vi "AlGaInPAs_v21e.vi"(2 "Debug Mode":bool, 3 "Elapsed Time(s)":dbl, 4 "State":enum16{"Edit", "Start", "Run", "End", "Idle"}(ring), 5 "Argument List In":string[](array[string])) -> (0 "Status Out":string, 1 "Argument List Out":string[](array[string]))   [LabVIEW 2011]
uses:
  high_level_proc/source_noDilute.ctl
  high_level_proc/source_noDilution.ctl
panel:
  in  "Zn bubbler":T1={"Dilution"=FALSE, "Calculated"=0, "MFC1 flow"=0.0, "MFC2 flow"=10.0, "MFC3 flow"=100.0, "Bubbler (main)"={"Flow"=0.0, "Prep"=FALSE, "Run"=FALSE, "Active"=FALSE, "Name"=""}} caption="Al" {"Bubbler (main)"."Flow" format="%.2f"; "MFC1 flow" format="%.4f"; "MFC3 flow" format="%.1f"; "MFC2 flow" format="%.2f"; "Calculated" items=["Flow", "MFC1", "MFC2", "MFC3"]}
  in  "Array":refnum<vi>[](array[refnum])
  in  "Al bubbler":T2 caption="Al" {"Flow" format="%.2f"}
  in  "Se bubbler":T1={"Dilution"=FALSE, "Calculated"=0, "MFC1 flow"=0.0, "MFC2 flow"=10.0, "MFC3 flow"=100.0, "Bubbler (main)"={"Flow"=0.0, "Prep"=FALSE, "Run"=FALSE, "Active"=FALSE, "Name"=""}} caption="Al" {"Bubbler (main)"."Flow" format="%.2f"; "MFC1 flow" format="%.4f"; "MFC3 flow" format="%.1f"; "MFC2 flow" format="%.2f"; "Calculated" items=["Flow", "MFC1", "MFC2", "MFC3"]}
  in  "P bubbler":T2 caption="Al" {"Flow" format="%.2f"}
  in  "As gas":T2 caption="Al" {"Flow" format="%.2f"}
  in  "P gas":T2 caption="Al" {"Flow" format="%.2f"}
  in  "In bubbler":T2 caption="Al" {"Flow" format="%.2f"}
  in  "Tab Control":T3(tab)
  out "Al Prep":bool caption="Pre-run"
  out "Al Run":bool caption="Run"
  out "Al Flow":dbl caption="Al Flow (0-100 sscm)" format="%.2f"
  out "Ga MFC1 flow":dbl caption="R1 (0-10 sscm)" format="%.4f"
  out "Ga MFC3 flow":dbl=100.0 caption="R3 (0-1000 sscm)" format="%.1f"
  out "Ga MFC2 flow":dbl=10.0 caption="R2 (0-100 sscm)" format="%.2f"
  out "Ga Calculated":u16(ring)=1 caption="Calculated" items=["Ga flow", "MFC1", "MFC2", "MFC3"]
  out "Ga Dilution":bool caption="Dilute"
  out "Ga Prep":bool caption="Pre-run"
  out "Ga Run":bool caption="Run"
  out "Ga Flow":dbl caption="Ga Flow (0-10 sscm)" format="%.2f"
  out "In Prep":bool caption="Pre-run"
  out "In Run":bool caption="Run"
  out "In Flow":dbl caption="In Flow (0-100 sscm)" format="%.2f"
  out "P gas Run":bool caption="Run"
  out "P gas Prep":bool caption="Pre-run"
  out "P gas Flow":dbl caption="PH3 Flow (0-100 sscm)" format="%.2f"
  out "As gas Prep":bool caption="Pre-run"
  out "As gas Run":bool caption="Run"
  out "As gas Flow":dbl caption="AsH3 Flow (0-10 sscm)" format="%.2f"
  out "P liq Prep":bool caption="Pre-run"
  out "P liq Run":bool caption="Run"
  out "P liq Flow":dbl caption="P bubbler Flow (0-100 sscm)" format="%.2f"
  out "Zn Flow":dbl caption="Zn Flow (0-10 sscm)" format="%.2f"
  out "Zn Run":bool caption="Run"
  out "Zn Prep":bool caption="Pre-run"
  out "Zn  Dilution":bool caption="Dilute"
  out "Zn Calculated":u16(ring)=1 caption="Calculated" items=["Ga flow", "MFC1", "MFC2", "MFC3"]
  out "Zn MFC2 flow":dbl=10.0 caption="R2 (0-100 sscm)" format="%.2f"
  out "Zn MFC3 flow":dbl=100.0 caption="R3 (0-1000 sscm)" format="%.1f"
  out "Zn MFC1 flow":dbl caption="R1 (0-10 sscm)" format="%.4f"
  out "Se MFC1 flow":dbl caption="R1 (0-10 sscm)" format="%.4f"
  out "Se MFC3 flow":dbl=100.0 caption="R3 (0-1000 sscm)" format="%.1f"
  out "Se MFC2 flow":dbl=10.0 caption="R2 (0-100 sscm)" format="%.2f"
  out "Se Calculated":u16(ring)=1 caption="Calculated" items=["Ga flow", "MFC1", "MFC2", "MFC3"]
  out "Se Dilution":bool caption="Dilute"
  out "Se Prep":bool caption="Pre-run"
  out "Se Run":bool caption="Run"
  out "Se Flow":dbl caption="Se Flow (0-10 sscm)" format="%.2f"
  in  "Ga bubbler":T1={"Dilution"=FALSE, "Calculated"=0, "MFC1 flow"=0.0, "MFC2 flow"=10.0, "MFC3 flow"=100.0, "Bubbler (main)"={"Flow"=0.0, "Prep"=FALSE, "Run"=FALSE, "Active"=FALSE, "Name"=""}} caption="Al" {"Bubbler (main)"."Flow" format="%.2f"; "MFC1 flow" format="%.4f"; "MFC3 flow" format="%.1f"; "MFC2 flow" format="%.2f"; "Calculated" items=["Flow", "MFC1", "MFC2", "MFC3"]}
  out "prep_done":bool
  out "run started":bool
  out "first":bool=TRUE
  out "total time":dbl
  out "is OK?":bool
  in  "prep_time":dbl
  in  "Cancel":bool
  in  "OK":bool
  out "tTotal(s) 2":dbl
  # "s"
  # "Add pre-run time to run time in editor."
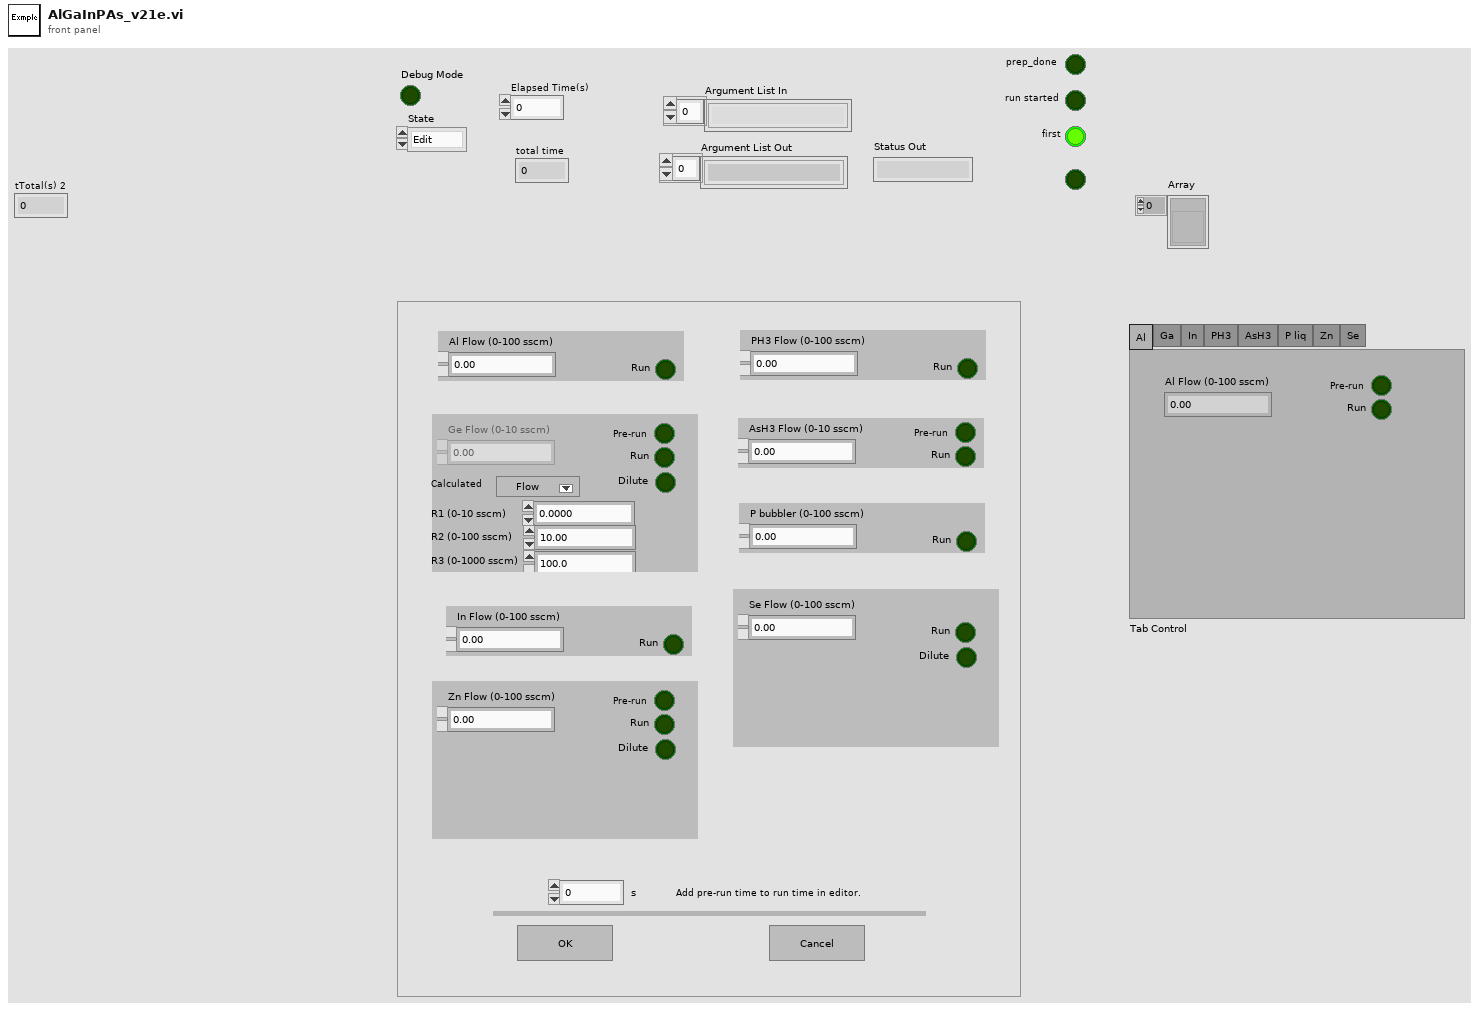
[diagram p1: front panel]
types:
  T1 = typedef "source_noDilute.ctl" = cluster{"Dilution":bool, "Calculated":u16, "MFC1 flow":dbl, "MFC2 flow":dbl, "MFC3 flow":dbl, "Bubbler (main)":T2}
  T2 = typedef "source_noDilution.ctl" = cluster{"Flow":dbl, "Prep":bool, "Run":bool, "Active":bool, "Name":string}
  T3 = enum32{"Al", "Ga", "In", "PH3", "AsH3", "P liq", "Zn", "Se"}
  T4 = enum16{"Discrete", "Continuous", "Instantaneous", "Finite"}
  T5 = enum32{"Invalid", "Default", "Floating", "Floating/Auto-Hide", "Modal"}
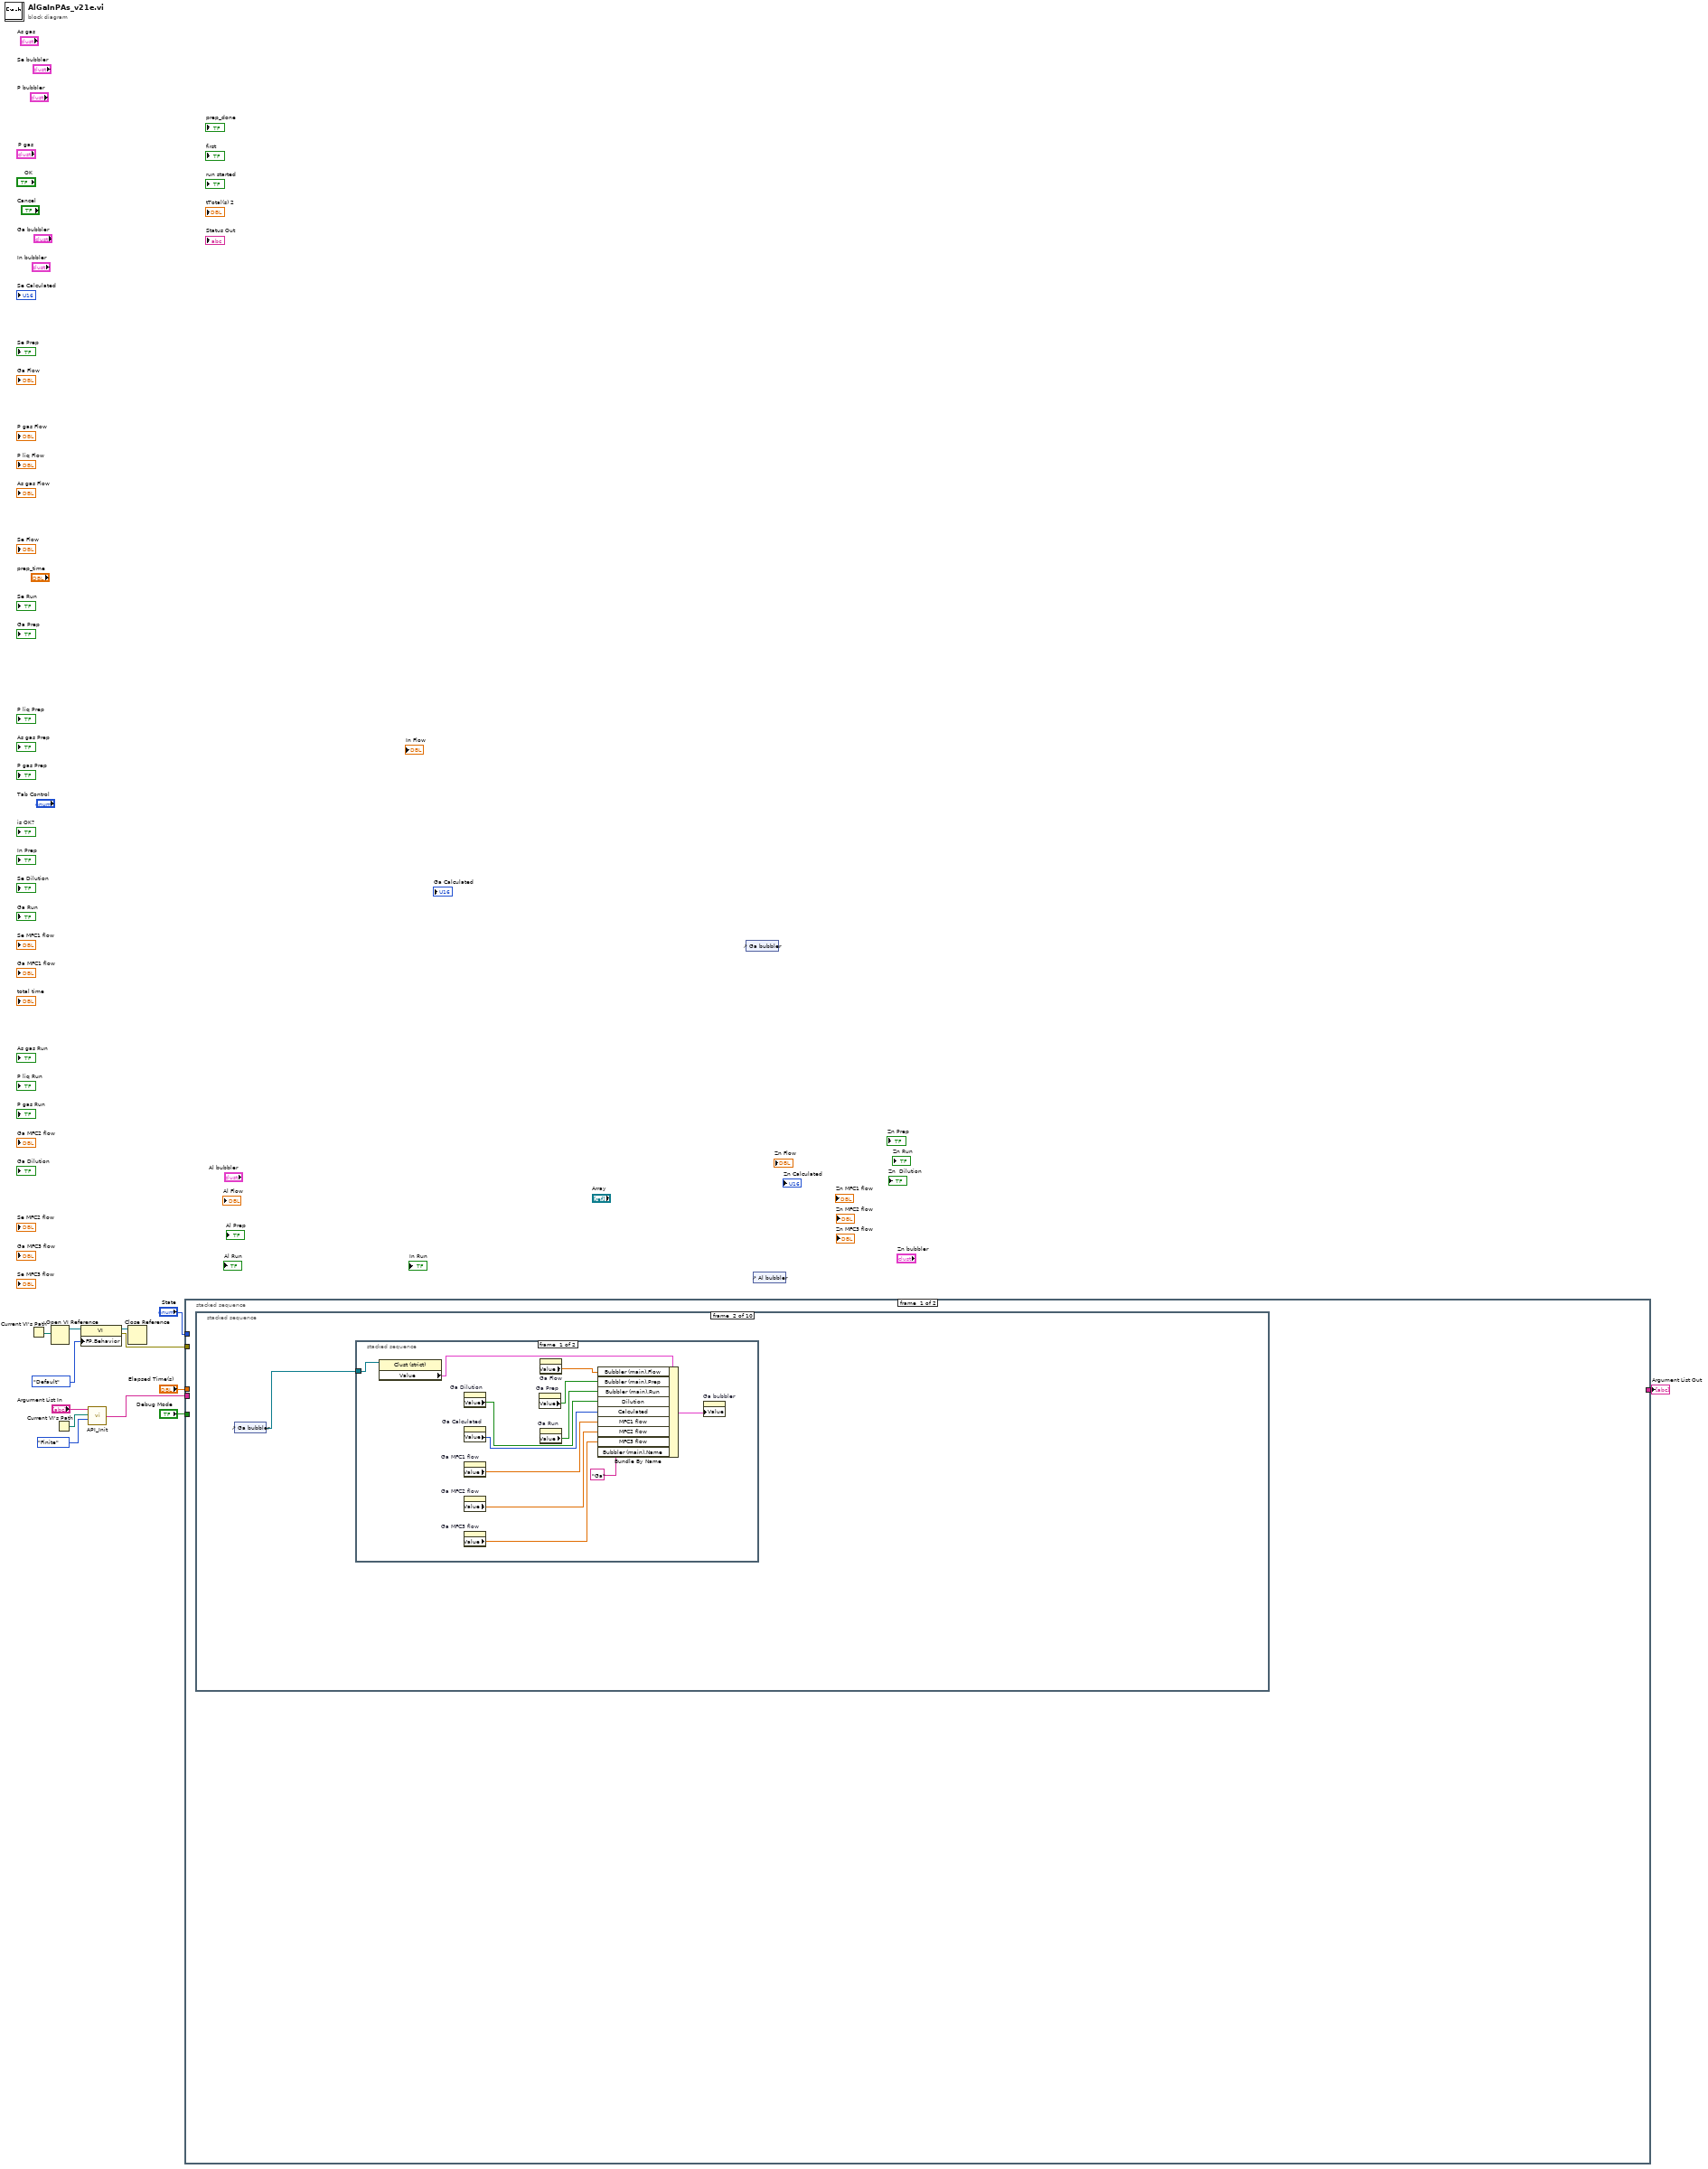
[diagram p0: block diagram]
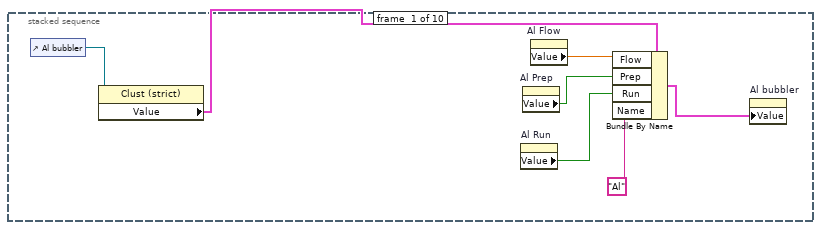
[diagram p2: hidden frame]
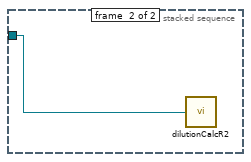
[diagram p3: hidden frame]
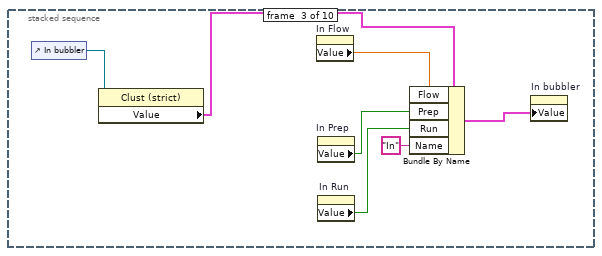
[diagram p4: hidden frame]
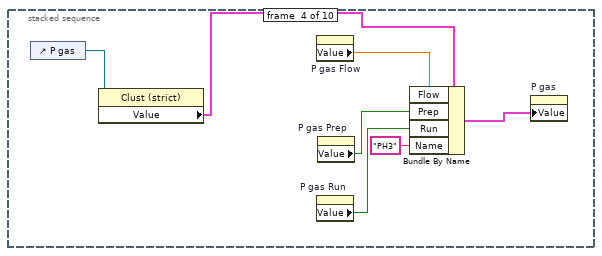
[diagram p5: hidden frame]
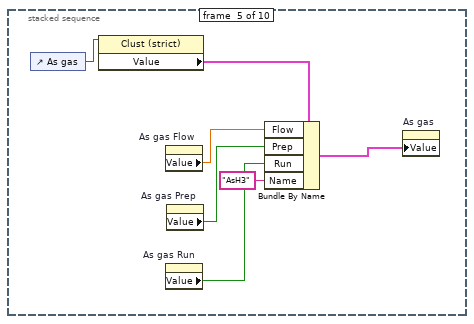
[diagram p6: hidden frame]
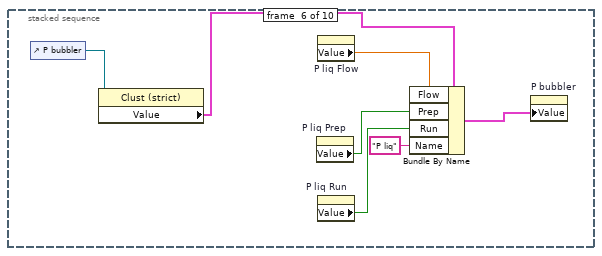
[diagram p7: hidden frame]
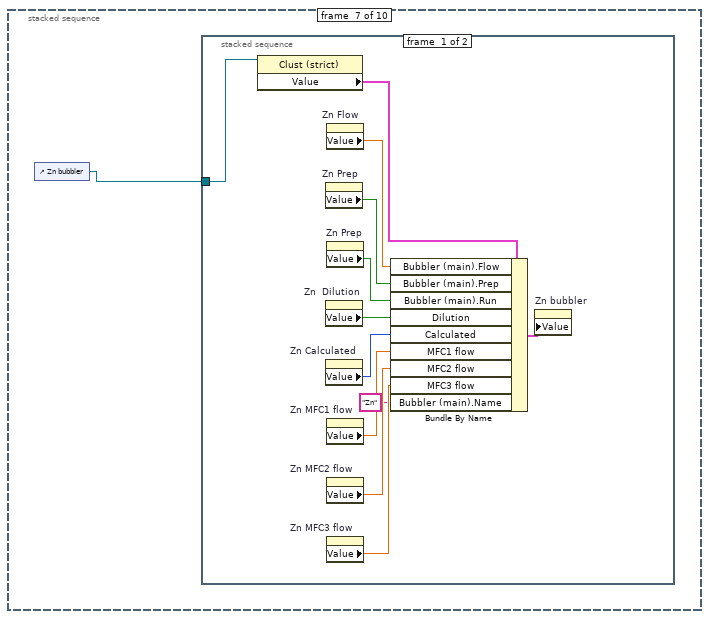
[diagram p8: hidden frame]
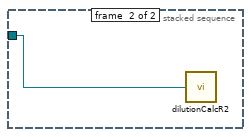
[diagram p9: hidden frame]
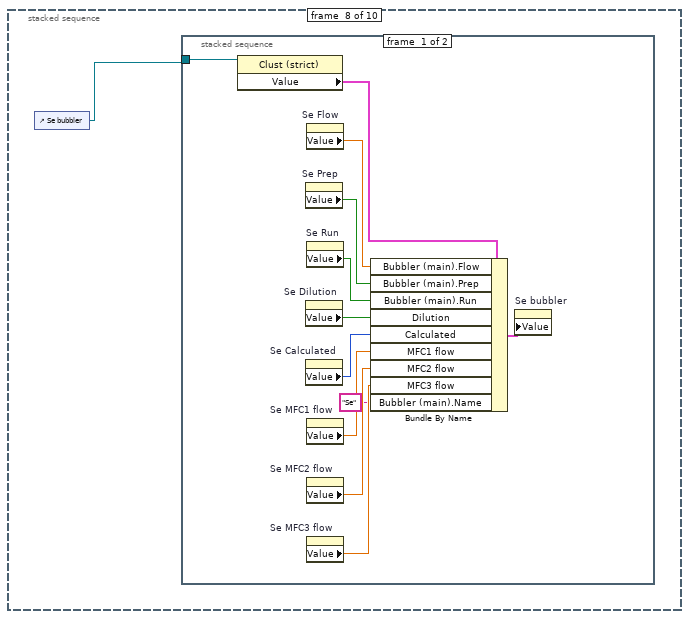
[diagram p10: hidden frame]
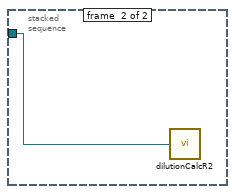
[diagram p11: hidden frame]
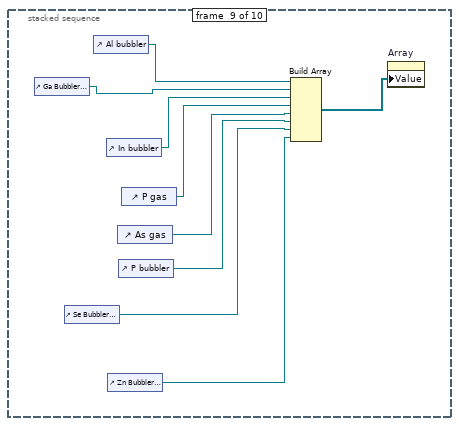
[diagram p12: hidden frame]
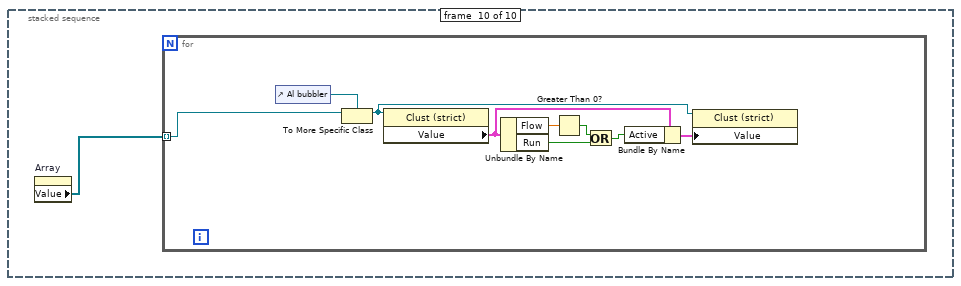
[diagram p13: hidden frame]
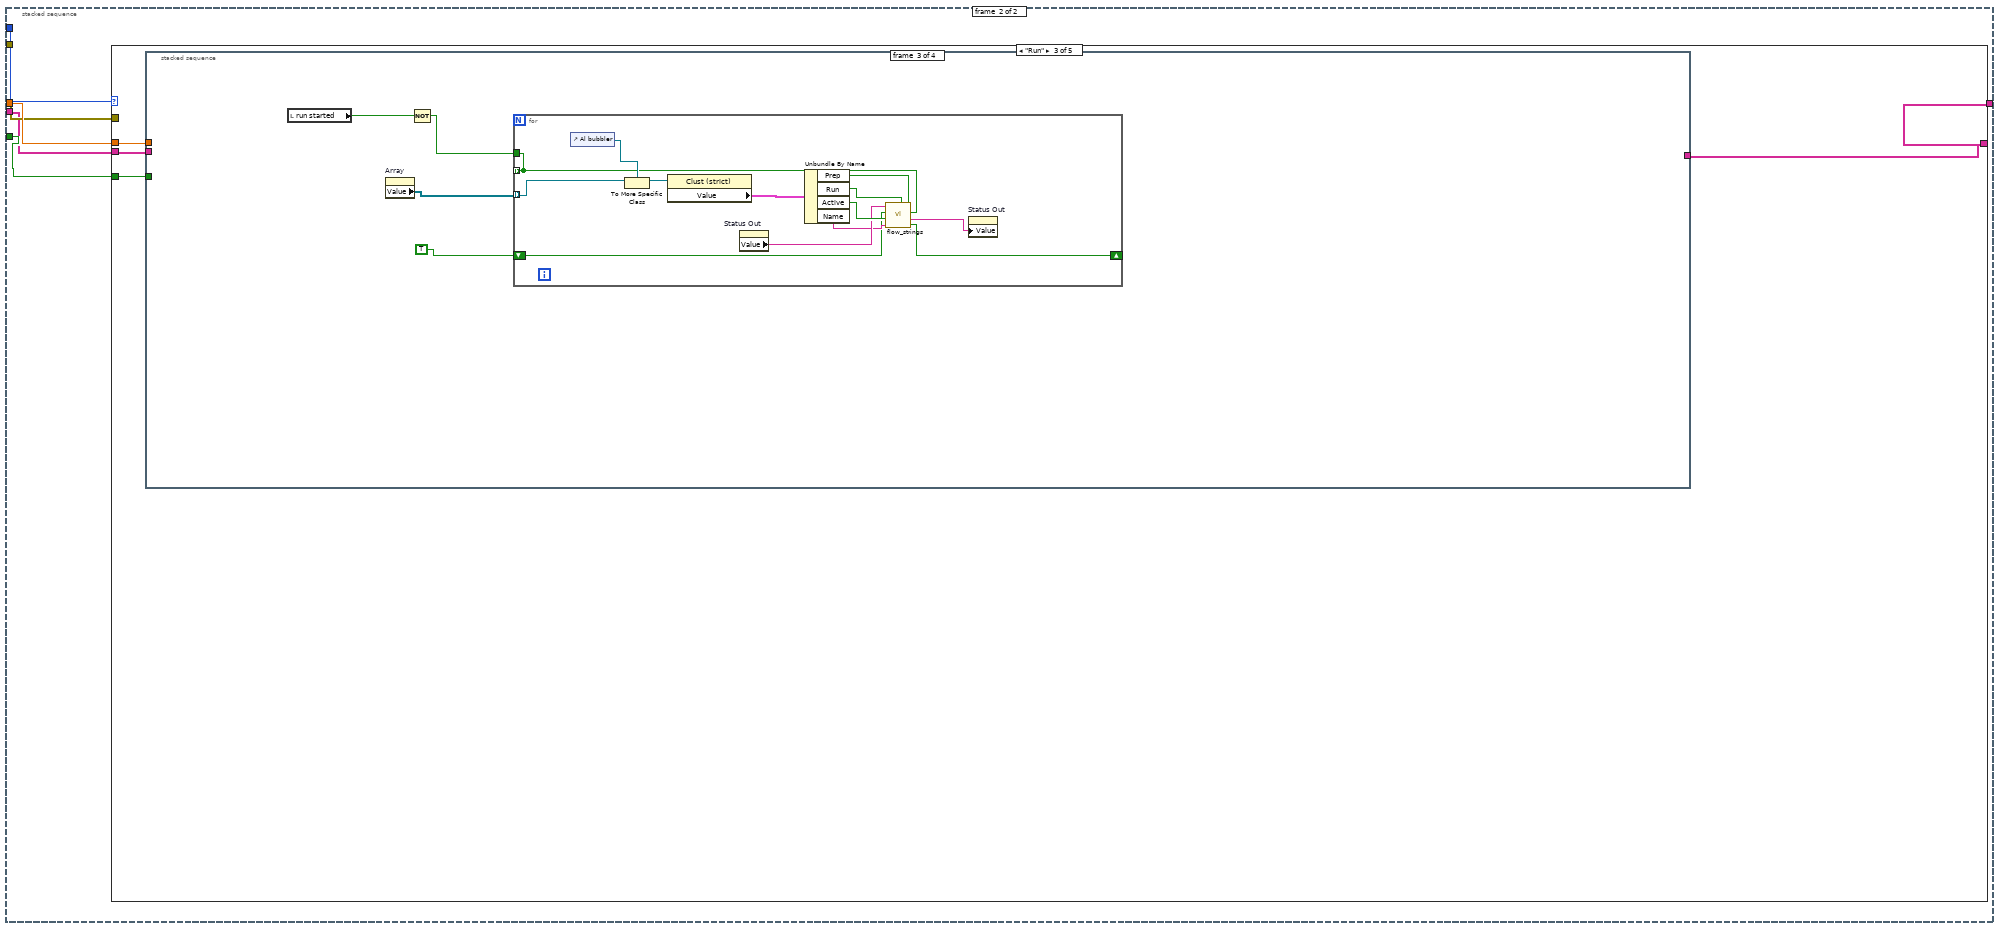
[diagram p14: hidden frame]
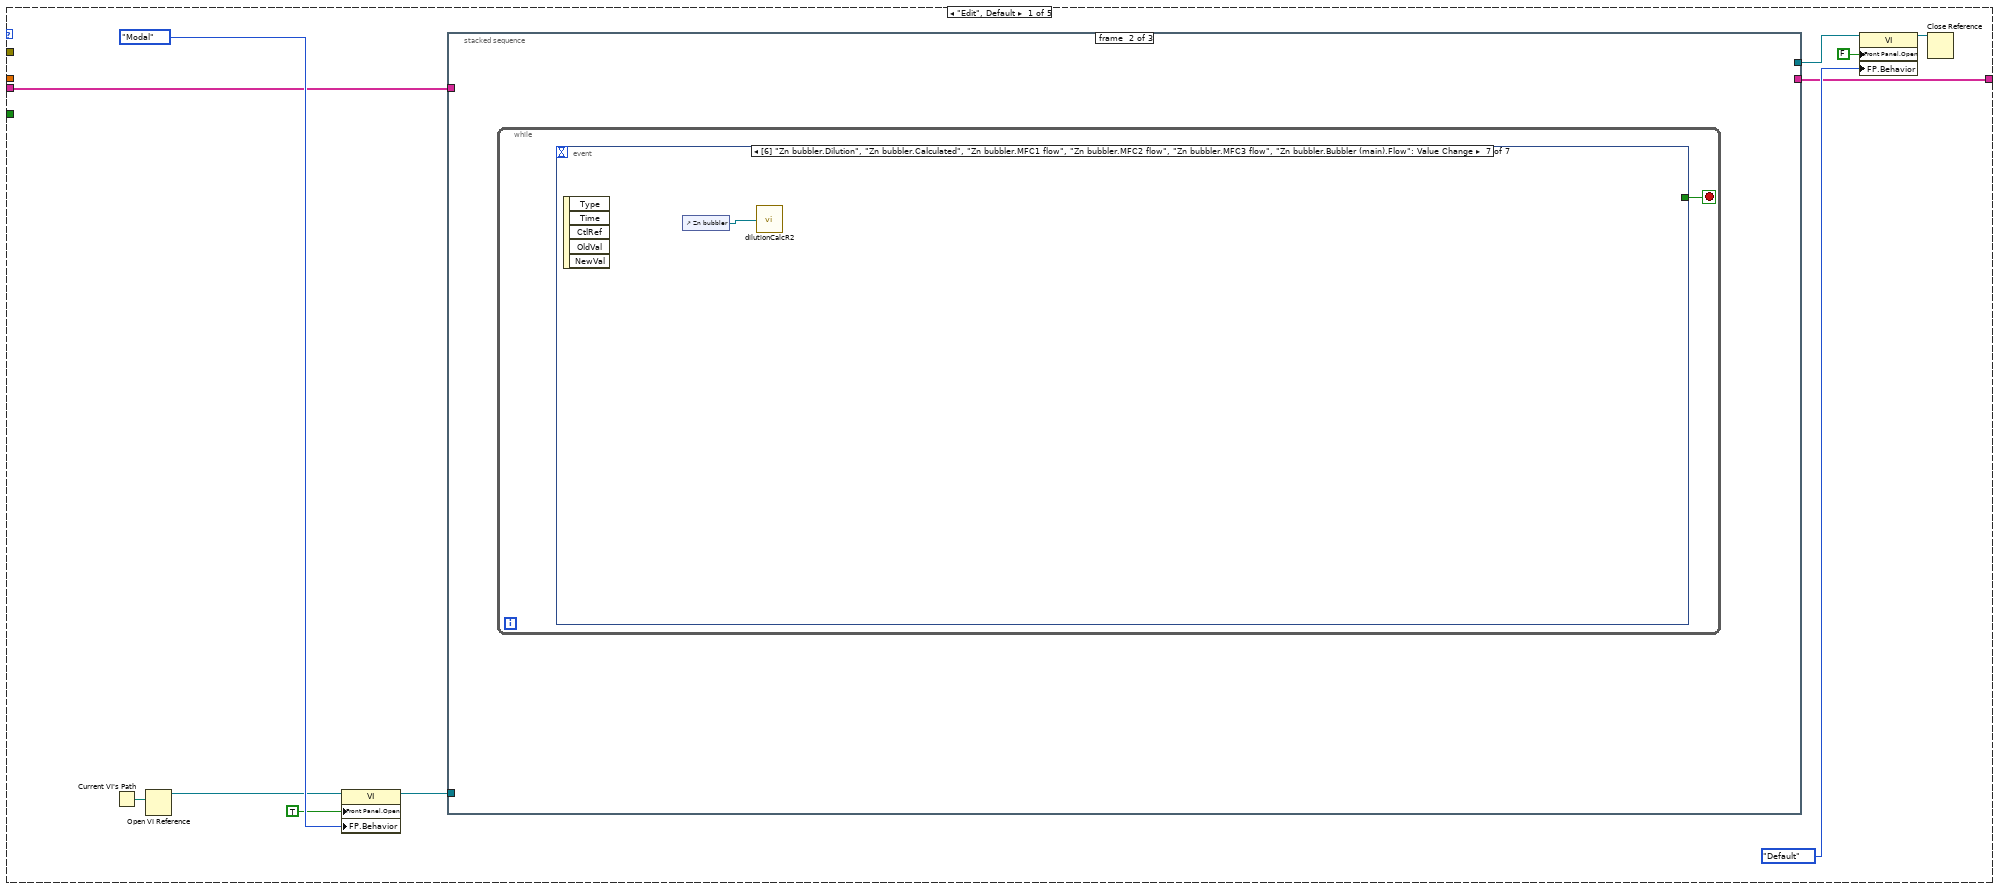
[diagram p15: hidden frame]
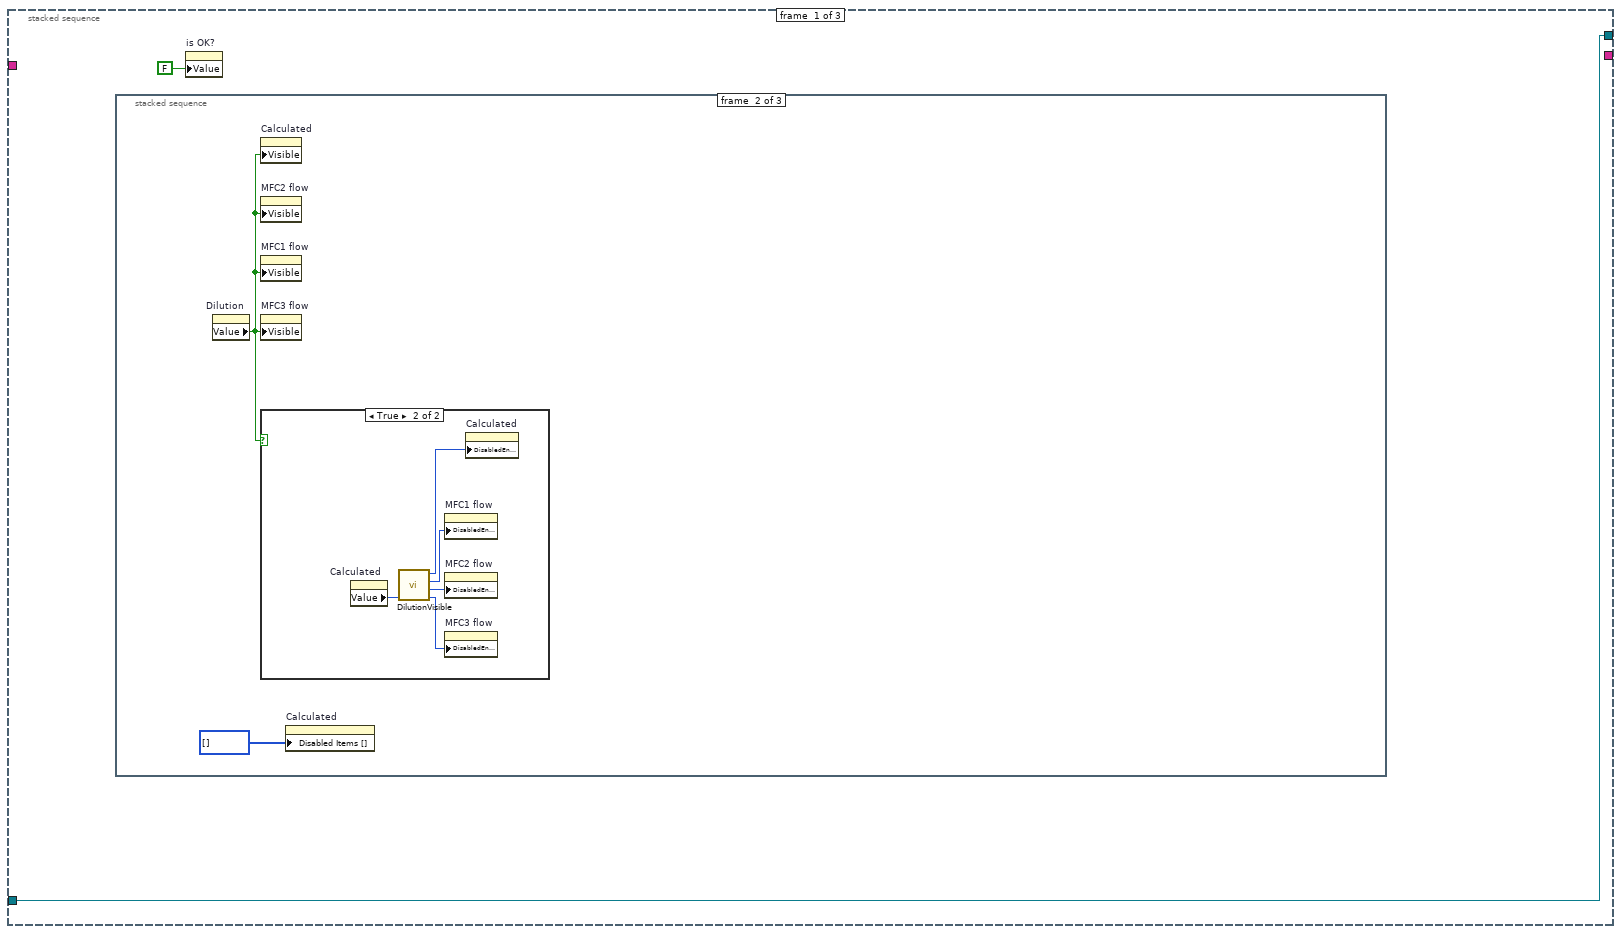
[diagram p16: hidden frame]
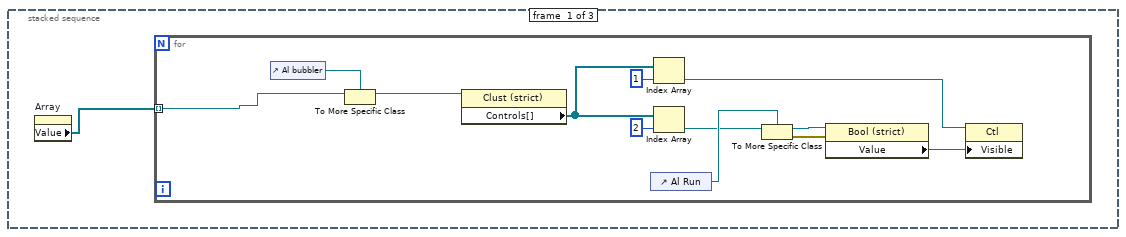
[diagram p17: hidden frame]
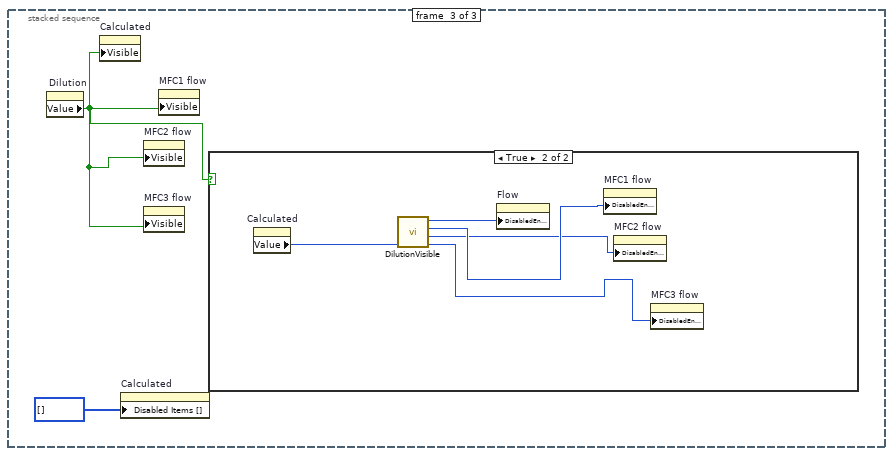
[diagram p19: hidden frame]
diagram:
  n1 = Current VI's Path() -> (path=w9:path)
  n2 = Open VI Reference(vi path=w9) -> (vi reference=w8:refnum<vi>)  [unwired: 1 in, 5 out]
  n3 = Current VI's Path() -> (path=w4:path)
  n4 = property class="VI"(reference=w8, "FP.Behavior"=T5."Default" ("Front Panel Window:Behavior")) -> (reference out=w6:refnum<vi>, error out=w5:errorcluster)  [unwired: 1 in]
  n5 = call "API_Init.vi"("API Mode"=T4."Finite", "VI Path"=w4, "Argument List In"="Argument List In") -> ("Argument List Out"=w1:string[])  [unwired: 1 in]
  n6 = Close Reference(reference=w6) -> ()  [unwired: 1 in, 1 out]
  n7 = stacked-sequence {
    tunnel: "State" -> [_ w115]
    tunnel: "Debug Mode" -> [_ w114]
    tunnel: "Elapsed Time(s)" -> [_ w113]
    tunnel: [_ w112] -> w10
    tunnel: w5 -> [_ w111]
    tunnel: w1 -> [_ w110]
    frame #0 {
      n8 = stacked-sequence {
        frame #0 {
          n9 = control-ref of="Al bubbler"() -> (w20:refnum<vi>)
          n10 = property class="Clust (strict)"(reference=w20) -> ("Value"=w19:T2)  [unwired: 1 in, 2 out]
          n11 = property on="Al Run" class="Bool (strict)"() -> ("Value"=w15:bool)  [unwired: 2 in, 2 out]
          n12 = property on="Al Prep" class="Bool (strict)"() -> ("Value"=w16:bool)  [unwired: 2 in, 2 out]
          n13 = property on="Al Flow" class="DigNum (strict)"() -> ("Value"=w18:dbl)  [unwired: 2 in, 2 out]
          n14 = Bundle By Name(cluster=w19, "Flow"=w18, "Prep"=w16, "Run"=w15, "Name"="Al") -> (w17:T2)
          n15 = property on="Al bubbler" class="Clust (strict)"("Value"=w17) -> ()  [unwired: 2 in, 2 out]
        }
        frame #1 {
          n16 = control-ref of="Ga bubbler"() -> (w21:refnum<vi>)
          n17 = stacked-sequence {
            tunnel: w21 -> [w25 w34]
            frame #0 {
              n18 = property class="Clust (strict)"(reference=w25) -> ("Value"=w24:T1)  [unwired: 1 in, 2 out]
              n19 = property on="Ga MFC1 flow" class="DigNum (strict)"() -> ("Value"=w31:dbl)  [unwired: 2 in, 2 out]
              n20 = property on="Ga MFC2 flow" class="DigNum (strict)"() -> ("Value"=w32:dbl)  [unwired: 2 in, 2 out]
              n21 = property on="Ga MFC3 flow" class="DigNum (strict)"() -> ("Value"=w33:dbl)  [unwired: 2 in, 2 out]
              n22 = property on="Ga Dilution" class="Bool (strict)"() -> ("Value"=w30:bool)  [unwired: 2 in, 2 out]
              n23 = property on="Ga Calculated" class="Ring (strict)"() -> ("Value"=w28:u16)  [unwired: 2 in, 2 out]
              n24 = property on="Ga Prep" class="Bool (strict)"() -> ("Value"=w27:bool)  [unwired: 2 in, 2 out]
              n25 = property on="Ga Flow" class="DigNum (strict)"() -> ("Value"=w26:dbl)  [unwired: 2 in, 2 out]
              n26 = property on="Ga Run" class="Bool (strict)"() -> ("Value"=w29:bool)  [unwired: 2 in, 2 out]
              n27 = Bundle By Name(cluster=w24, "Bubbler (main).Flow"=w26, "Bubbler (main).Prep"=w27, "Bubbler (main).Run"=w29, "Dilution"=w30, "Calculated"=w28, "MFC1 flow"=w31, "MFC2 flow"=w32, "MFC3 flow"=w33, "Bubbler (main).Name"="Ga") -> (w22:T1)
              n28 = property on="Ga bubbler" class="Clust (strict)"("Value"=w22) -> ()  [unwired: 2 in, 2 out]
            }
            frame #1 {
              n29 = call "dilutionCalcR2.vi"("Clust Refnum"=w34) -> ()
            }
          }
        }
        frame #2 {
          n30 = control-ref of="In bubbler"() -> (w36:refnum<vi>)
          n31 = property class="Clust (strict)"(reference=w36) -> ("Value"=w37:T2)  [unwired: 1 in, 2 out]
          n32 = property on="In Flow" class="DigNum (strict)"() -> ("Value"=w38:dbl)  [unwired: 2 in, 2 out]
          n33 = property on="In Prep" class="Bool (strict)"() -> ("Value"=w40:bool)  [unwired: 2 in, 2 out]
          n34 = property on="In Run" class="Bool (strict)"() -> ("Value"=w41:bool)  [unwired: 2 in, 2 out]
          n35 = Bundle By Name(cluster=w37, "Flow"=w38, "Prep"=w40, "Run"=w41, "Name"="In") -> (w39:T2)
          n36 = property on="In bubbler" class="Clust (strict)"("Value"=w39) -> ()  [unwired: 2 in, 2 out]
        }
        frame #3 {
          n37 = control-ref of="P gas"() -> (w43:refnum<vi>)
          n38 = property class="Clust (strict)"(reference=w43) -> ("Value"=w44:T2)  [unwired: 1 in, 2 out]
          n39 = property on="P gas Flow" class="DigNum (strict)"() -> ("Value"=w45:dbl)  [unwired: 2 in, 2 out]
          n40 = property on="P gas Run" class="Bool (strict)"() -> ("Value"=w48:bool)  [unwired: 2 in, 2 out]
          n41 = property on="P gas Prep" class="Bool (strict)"() -> ("Value"=w47:bool)  [unwired: 2 in, 2 out]
          n42 = Bundle By Name(cluster=w44, "Flow"=w45, "Prep"=w47, "Run"=w48, "Name"="PH3") -> (w46:T2)
          n43 = property on="P gas" class="Clust (strict)"("Value"=w46) -> ()  [unwired: 2 in, 2 out]
        }
        frame #4 {
          n44 = control-ref of="As gas"() -> (w51:refnum<vi>)
          n45 = property class="Clust (strict)"(reference=w51) -> ("Value"=w50:T2)  [unwired: 1 in, 2 out]
          n46 = property on="As gas Flow" class="DigNum (strict)"() -> ("Value"=w53:dbl)  [unwired: 2 in, 2 out]
          n47 = property on="As gas Run" class="Bool (strict)"() -> ("Value"=w55:bool)  [unwired: 2 in, 2 out]
          n48 = property on="As gas Prep" class="Bool (strict)"() -> ("Value"=w54:bool)  [unwired: 2 in, 2 out]
          n49 = Bundle By Name(cluster=w50, "Flow"=w53, "Prep"=w54, "Run"=w55, "Name"="AsH3") -> (w52:T2)
          n50 = property on="As gas" class="Clust (strict)"("Value"=w52) -> ()  [unwired: 2 in, 2 out]
        }
        frame #5 {
          n51 = control-ref of="P bubbler"() -> (w57:refnum<vi>)
          n52 = property class="Clust (strict)"(reference=w57) -> ("Value"=w58:T2)  [unwired: 1 in, 2 out]
          n53 = property on="P liq Prep" class="Bool (strict)"() -> ("Value"=w61:bool)  [unwired: 2 in, 2 out]
          n54 = property on="P liq Flow" class="DigNum (strict)"() -> ("Value"=w60:dbl)  [unwired: 2 in, 2 out]
          n55 = property on="P liq Run" class="Bool (strict)"() -> ("Value"=w62:bool)  [unwired: 2 in, 2 out]
          n56 = Bundle By Name(cluster=w58, "Flow"=w60, "Prep"=w61, "Run"=w62, "Name"="P liq") -> (w59:T2)
          n57 = property on="P bubbler" class="Clust (strict)"("Value"=w59) -> ()  [unwired: 2 in, 2 out]
        }
        frame #6 {
          n58 = control-ref of="Zn bubbler"() -> (w63:refnum<vi>)
          n59 = stacked-sequence {
            tunnel: w63 -> [w65 w76]
            frame #0 {
              n60 = property class="Clust (strict)"(reference=w65) -> ("Value"=w66:T1)  [unwired: 1 in, 2 out]
              n61 = property on="Zn Prep" class="Bool (strict)"() -> ("Value"=w69:bool)  [unwired: 2 in, 2 out]
              n62 = property on="Zn  Dilution" class="Bool (strict)"() -> ("Value"=w71:bool)  [unwired: 2 in, 2 out]
              n63 = property on="Zn Calculated" class="Ring (strict)"() -> ("Value"=w72:u16)  [unwired: 2 in, 2 out]
              n64 = property on="Zn Flow" class="DigNum (strict)"() -> ("Value"=w68:dbl)  [unwired: 2 in, 2 out]
              n65 = property on="Zn Prep" class="Bool (strict)"() -> ("Value"=w70:bool)  [unwired: 2 in, 2 out]
              n66 = property on="Zn MFC1 flow" class="DigNum (strict)"() -> ("Value"=w73:dbl)  [unwired: 2 in, 2 out]
              n67 = property on="Zn MFC2 flow" class="DigNum (strict)"() -> ("Value"=w74:dbl)  [unwired: 2 in, 2 out]
              n68 = property on="Zn MFC3 flow" class="DigNum (strict)"() -> ("Value"=w75:dbl)  [unwired: 2 in, 2 out]
              n69 = Bundle By Name(cluster=w66, "Bubbler (main).Flow"=w68, "Bubbler (main).Prep"=w69, "Bubbler (main).Run"=w70, "Dilution"=w71, "Calculated"=w72, "MFC1 flow"=w73, "MFC2 flow"=w74, "MFC3 flow"=w75, "Bubbler (main).Name"="Zn") -> (w67:T1)
              n70 = property on="Zn bubbler" class="Clust (strict)"("Value"=w67) -> ()  [unwired: 2 in, 2 out]
            }
            frame #1 {
              n71 = call "dilutionCalcR2.vi"("Clust Refnum"=w76) -> ()
            }
          }
        }
        frame #7 {
          n72 = control-ref of="Se bubbler"() -> (w77:refnum<vi>)
          n73 = stacked-sequence {
            tunnel: w77 -> [w79 w90]
            frame #0 {
              n74 = property class="Clust (strict)"(reference=w79) -> ("Value"=w80:T1)  [unwired: 1 in, 2 out]
              n75 = property on="Se Prep" class="Bool (strict)"() -> ("Value"=w83:bool)  [unwired: 2 in, 2 out]
              n76 = property on="Se Dilution" class="Bool (strict)"() -> ("Value"=w85:bool)  [unwired: 2 in, 2 out]
              n77 = property on="Se Calculated" class="Ring (strict)"() -> ("Value"=w86:u16)  [unwired: 2 in, 2 out]
              n78 = property on="Se Flow" class="DigNum (strict)"() -> ("Value"=w82:dbl)  [unwired: 2 in, 2 out]
              n79 = property on="Se Run" class="Bool (strict)"() -> ("Value"=w84:bool)  [unwired: 2 in, 2 out]
              n80 = property on="Se MFC1 flow" class="DigNum (strict)"() -> ("Value"=w87:dbl)  [unwired: 2 in, 2 out]
              n81 = property on="Se MFC2 flow" class="DigNum (strict)"() -> ("Value"=w88:dbl)  [unwired: 2 in, 2 out]
              n82 = property on="Se MFC3 flow" class="DigNum (strict)"() -> ("Value"=w89:dbl)  [unwired: 2 in, 2 out]
              n83 = Bundle By Name(cluster=w80, "Bubbler (main).Flow"=w82, "Bubbler (main).Prep"=w83, "Bubbler (main).Run"=w84, "Dilution"=w85, "Calculated"=w86, "MFC1 flow"=w87, "MFC2 flow"=w88, "MFC3 flow"=w89, "Bubbler (main).Name"="Se") -> (w81:T1)
              n84 = property on="Se bubbler" class="Clust (strict)"("Value"=w81) -> ()  [unwired: 2 in, 2 out]
            }
            frame #1 {
              n85 = call "dilutionCalcR2.vi"("Clust Refnum"=w90) -> ()
            }
          }
        }
        frame #8 {
          n86 = control-ref of="Ga Bubbler (main)"() -> (w93:refnum<vi>)
          n87 = control-ref of="Se Bubbler (main)"() -> (w92:refnum<vi>)
          n88 = control-ref of="Al bubbler"() -> (w98:refnum<vi>)
          n89 = control-ref of="In bubbler"() -> (w97:refnum<vi>)
          n90 = control-ref of="Zn Bubbler (main)"() -> (w91:refnum<vi>)
          n91 = control-ref of="As gas"() -> (w95:refnum<vi>)
          n92 = control-ref of="P bubbler"() -> (w94:refnum<vi>)
          n93 = control-ref of="P gas"() -> (w96:refnum<vi>)
          n94 = Build Array(w98, w93, w97, w96, w95, w94, w92, w91) -> (w99:refnum<vi>[])
          n95 = property on="Array" class="Arr (strict)"("Value"=w99) -> ()  [unwired: 2 in, 2 out]
        }
        frame #9 {
          n96 = property on="Array" class="Arr (strict)"() -> ("Value"=w100:refnum<vi>[])  [unwired: 2 in, 2 out]
          n97 = for {
            tunnel: w100 -> [w108] mode=indexing
            n98 = control-ref of="Al bubbler"() -> (w109:refnum<vi>)
            n99 = To More Specific Class(target class=w109, reference=w108) -> (specific class reference=w104:refnum<vi>)  [unwired: 1 in, 1 out]
            n100 = property class="Clust (strict)"(reference=w104) -> ("Value"=w103:T2)  [unwired: 1 in, 2 out]
            n101 = Unbundle By Name(w103) -> ("Flow"=w107:dbl, "Run"=w105:bool)
            n102 = Greater Than 0?(x=w107) -> (x > 0?=w106:bool)
            n103 = Or(x=w106, y=w105) -> (x .or. y?=w101:bool)
            n104 = Bundle By Name(cluster=w103, "Active"=w101) -> (w102:T2)
            n105 = property class="Clust (strict)"(reference=w104, "Value"=w102) -> ()  [unwired: 1 in, 2 out]
          }
        }
      }
    }
    frame #1 {
      n106 = case shown="\"Run\"" w115 {
        tunnel: w114 -> [_ w229 w248 _ _]
        tunnel: w113 -> [_ _ w249 _ _]
        tunnel: w110 -> [w117 w234 w247 w300 w301]
        tunnel: [w116 w233 w246 w300 w301] -> w112
        tunnel: w111 -> [_ _ _ _ _]
        frame "Edit", Default {
          n107 = Current VI's Path() -> (path=w122:path)
          n108 = Open VI Reference(vi path=w122) -> (vi reference=w121:refnum<vi>)  [unwired: 1 in, 5 out]
          n109 = property class="VI"(reference=w121, "Front Panel.Open"=TRUE ("Front Panel Window:Open"), "FP.Behavior"=T5."Modal" ("Front Panel Window:Behavior")) -> (reference out=w120:refnum<vi>)  [unwired: 1 in, 1 out]
          n110 = stacked-sequence {
            tunnel: w117 -> [_ _ w224]
            tunnel: w120 -> [w128 _ _]
            tunnel: [w128 _ _] -> w124
            tunnel: [_ _ w225] -> w116
            frame #0 {
              n111 = stacked-sequence {
                frame #0 {
                  n112 = property on="Array" class="Arr (strict)"() -> ("Value"=w129:refnum<vi>[])  [unwired: 2 in, 2 out]
                  n113 = for {
                    tunnel: w129 -> [w130] mode=indexing
                    n114 = control-ref of="Al bubbler"() -> (w131:refnum<vi>)
                    n115 = To More Specific Class(target class=w131, reference=w130) -> (specific class reference=w139:refnum<vi>)  [unwired: 1 in, 1 out]
                    n116 = property class="Clust (strict)"(reference=w139) -> ("Controls[]"=w138:refnum<vi>[])  [unwired: 1 in, 2 out]
                    n117 = control-ref of="Al Run"() -> (w136:refnum<vi>)
                    n118 = Index Array(array=w138, index=1) -> (element=w140:refnum<vi>)
                    n119 = Index Array(array=w138, index=2) -> (element=w135:refnum<vi>)
                    n120 = To More Specific Class(target class=w136, reference=w135) -> (specific class reference=w134:refnum<vi>, error out=w133:errorcluster)  [unwired: 1 in]
                    n121 = property class="Bool (strict)"(reference=w134, error in=w133) -> ("Value"=w132:bool)  [unwired: 2 out]
                    n122 = property class="Ctl"(reference=w140, "Visible"=w132) -> ()  [unwired: 1 in, 2 out]
                  }
                }
                frame #1 {
                  n123 = property on="Dilution" class="Bool (strict)"() -> ("Value"=w143:bool)  [unwired: 2 in, 2 out]
                  n124 = property on="Calculated" class="Ring (strict)"("Visible"=w143) -> ()  [unwired: 2 in, 2 out]
                  n125 = property on="MFC2 flow" class="DigNum (strict)"("Visible"=w143) -> ()  [unwired: 2 in, 2 out]
                  n126 = property on="MFC1 flow" class="DigNum (strict)"("Visible"=w143) -> ()  [unwired: 2 in, 2 out]
                  n127 = property on="MFC3 flow" class="DigNum (strict)"("Visible"=w143) -> ()  [unwired: 2 in, 2 out]
                  n128 = case shown="True" w143 {
                    frame False {
                    }
                    frame True {
                      n129 = property on="Calculated" class="Ring (strict)"() -> ("Value"=w145:u16)  [unwired: 2 in, 2 out]
                      n130 = call "DilutionVisible.vi"("calculated"=w145) -> ("MFC3"=w148:u16, "MFC2"=w147:u16, "MFC1"=w146:u16, "flow"=w144:u16)  [unwired: 3 in]
                      n131 = property on="MFC1 flow" class="DigNum (strict)"("DisabledEnum"=w146) -> ()  [unwired: 2 in, 2 out]
                      n132 = property on="MFC2 flow" class="DigNum (strict)"("DisabledEnum"=w147) -> ()  [unwired: 2 in, 2 out]
                      n133 = property on="MFC3 flow" class="DigNum (strict)"("DisabledEnum"=w148) -> ()  [unwired: 2 in, 2 out]
                      n134 = property on="Calculated" class="Ring (strict)"("DisabledEnum"=w144) -> ()  [unwired: 2 in, 2 out]
                    }
                  }
                  n135 = property on="Calculated" class="Ring (strict)"("Disabled Items []"=i32[] []) -> ()  [unwired: 2 in, 2 out]
                }
                frame #2 {
                  n136 = property on="Dilution" class="Bool (strict)"() -> ("Value"=w149:bool)  [unwired: 2 in, 2 out]
                  n137 = property on="Calculated" class="Ring (strict)"("Visible"=w149) -> ()  [unwired: 2 in, 2 out]
                  n138 = property on="Calculated" class="Ring (strict)"("Disabled Items []"=i32[] []) -> ()  [unwired: 2 in, 2 out]
                  n139 = property on="MFC2 flow" class="DigNum (strict)"("Visible"=w149) -> ()  [unwired: 2 in, 2 out]
                  n140 = property on="MFC3 flow" class="DigNum (strict)"("Visible"=w149) -> ()  [unwired: 2 in, 2 out]
                  n141 = property on="MFC1 flow" class="DigNum (strict)"("Visible"=w149) -> ()  [unwired: 2 in, 2 out]
                  n142 = case shown="True" w149 {
                    frame False {
                    }
                    frame True {
                      n143 = property on="Calculated" class="Ring (strict)"() -> ("Value"=w154:u16)  [unwired: 2 in, 2 out]
                      n144 = call "DilutionVisible.vi"("calculated"=w154) -> ("MFC3"=w152:u16, "MFC2"=w151:u16, "MFC1"=w153:u16, "flow"=w155:u16)  [unwired: 3 in]
                      n145 = property on="Flow" class="DigNum (strict)"("DisabledEnum"=w155) -> ()  [unwired: 2 in, 2 out]
                      n146 = property on="MFC1 flow" class="DigNum (strict)"("DisabledEnum"=w153) -> ()  [unwired: 2 in, 2 out]
                      n147 = property on="MFC2 flow" class="DigNum (strict)"("DisabledEnum"=w151) -> ()  [unwired: 2 in, 2 out]
                      n148 = property on="MFC3 flow" class="DigNum (strict)"("DisabledEnum"=w152) -> ()  [unwired: 2 in, 2 out]
                    }
                  }
                }
              }
              n149 = property on="is OK?" class="Bool (strict)"("Value"=FALSE ("is OK?")) -> ()  [unwired: 2 in, 2 out]
            }
            frame #1 {
              n150 = while {
                stop <- w156 stop-if-true
                n151 = event shown="[6] \"Zn bubbler.Dilution\", \"Zn bubbler.Calculated\", \"Zn bubbler.MFC1 flow\", \"Zn bubbler.MFC2 flow\", \"Zn bubbler.MFC3 flow\", \"Zn bubbler.Bubbler (main).Flow\": Value Change" {
                  selector: _ -> [_ _ _ _ _ _ _]
                  dyn-events: _ -> [_ _ _ _ _ _ _]
                  timeout: _ -> [_ _ _ _ _ _ _]
                  tunnel: [_ TRUE _ TRUE _ _ _] -> w156
                  event Timeout {
                    n152 = event-data() -> ()  [unwired: 1 in, 2 out]
                  }
                  event "OK": Value Change {
                    n153 = event-data() -> ()  [unwired: 1 in, 5 out]
                    n154 = stacked-sequence {
                      frame #0 {
                        n155 = property on="Al bubbler" class="Clust (strict)"() -> ("Value"=w159:T2)  [unwired: 2 in, 2 out]
                        n156 = Unbundle By Name(w159) -> ("Prep"=w162:bool, "Run"=w161:bool, "Flow"=w160:dbl)
                        n157 = property on="Al Prep" class="Bool (strict)"("Value"=w162) -> ()  [unwired: 2 in, 2 out]
                        n158 = property on="Al Run" class="Bool (strict)"("Value"=w161) -> ()  [unwired: 2 in, 2 out]
                        n159 = property on="Al Flow" class="DigNum (strict)"("Value"=w160) -> ()  [unwired: 2 in, 2 out]
                      }
                      frame #1 {
                        n160 = property on="Ga bubbler" class="Clust (strict)"() -> ("Value"=w171:T1)  [unwired: 2 in, 2 out]
                        n161 = Unbundle By Name(w171) -> ("Bubbler (main).Prep"=w170:bool, "Bubbler (main).Run"=w169:bool, "Bubbler (main).Flow"=w168:dbl, "Dilution"=w167:bool, "Calculated"=w166:u16, "MFC1 flow"=w165:dbl, "MFC2 flow"=w164:dbl, "MFC3 flow"=w163:dbl)
                        n162 = property on="Ga Prep" class="Bool (strict)"("Value"=w170) -> ()  [unwired: 2 in, 2 out]
                        n163 = property on="Ga Run" class="Bool (strict)"("Value"=w169) -> ()  [unwired: 2 in, 2 out]
                        n164 = property on="Ga Flow" class="DigNum (strict)"("Value"=w168) -> ()  [unwired: 2 in, 2 out]
                        n165 = property on="Ga Dilution" class="Bool (strict)"("Value"=w167) -> ()  [unwired: 2 in, 2 out]
                        n166 = property on="Ga Calculated" class="Ring (strict)"("Value"=w166) -> ()  [unwired: 2 in, 2 out]
                        n167 = property on="Ga MFC1 flow" class="DigNum (strict)"("Value"=w165) -> ()  [unwired: 2 in, 2 out]
                        n168 = property on="Ga MFC2 flow" class="DigNum (strict)"("Value"=w164) -> ()  [unwired: 2 in, 2 out]
                        n169 = property on="Ga MFC3 flow" class="DigNum (strict)"("Value"=w163) -> ()  [unwired: 2 in, 2 out]
                      }
                      frame #2 {
                        n170 = property on="In bubbler" class="Clust (strict)"() -> ("Value"=w175:T2)  [unwired: 2 in, 2 out]
                        n171 = Unbundle By Name(w175) -> ("Prep"=w174:bool, "Run"=w173:bool, "Flow"=w172:dbl)
                        n172 = property on="In Prep" class="Bool (strict)"("Value"=w174) -> ()  [unwired: 2 in, 2 out]
                        n173 = property on="In Run" class="Bool (strict)"("Value"=w173) -> ()  [unwired: 2 in, 2 out]
                        n174 = property on="In Flow" class="DigNum (strict)"("Value"=w172) -> ()  [unwired: 2 in, 2 out]
                      }
                      frame #3 {
                        n175 = property on="P gas" class="Clust (strict)"() -> ("Value"=w179:T2)  [unwired: 2 in, 2 out]
                        n176 = Unbundle By Name(w179) -> ("Prep"=w178:bool, "Run"=w177:bool, "Flow"=w176:dbl)
                        n177 = property on="P gas Prep" class="Bool (strict)"("Value"=w178) -> ()  [unwired: 2 in, 2 out]
                        n178 = property on="P gas Run" class="Bool (strict)"("Value"=w177) -> ()  [unwired: 2 in, 2 out]
                        n179 = property on="P gas Flow" class="DigNum (strict)"("Value"=w176) -> ()  [unwired: 2 in, 2 out]
                      }
                      frame #4 {
                        n180 = property on="As gas" class="Clust (strict)"() -> ("Value"=w183:T2)  [unwired: 2 in, 2 out]
                        n181 = Unbundle By Name(w183) -> ("Prep"=w182:bool, "Run"=w181:bool, "Flow"=w180:dbl)
                        n182 = property on="As gas Prep" class="Bool (strict)"("Value"=w182) -> ()  [unwired: 2 in, 2 out]
                        n183 = property on="As gas Run" class="Bool (strict)"("Value"=w181) -> ()  [unwired: 2 in, 2 out]
                        n184 = property on="As gas Flow" class="DigNum (strict)"("Value"=w180) -> ()  [unwired: 2 in, 2 out]
                      }
                      frame #5 {
                        n185 = property on="P bubbler" class="Clust (strict)"() -> ("Value"=w187:T2)  [unwired: 2 in, 2 out]
                        n186 = Unbundle By Name(w187) -> ("Prep"=w186:bool, "Run"=w185:bool, "Flow"=w184:dbl)
                        n187 = property on="P liq Prep" class="Bool (strict)"("Value"=w186) -> ()  [unwired: 2 in, 2 out]
                        n188 = property on="P liq Run" class="Bool (strict)"("Value"=w185) -> ()  [unwired: 2 in, 2 out]
                        n189 = property on="P liq Flow" class="DigNum (strict)"("Value"=w184) -> ()  [unwired: 2 in, 2 out]
                      }
                      frame #6 {
                        n190 = property on="Zn bubbler" class="Clust (strict)"() -> ("Value"=w196:T1)  [unwired: 2 in, 2 out]
                        n191 = Unbundle By Name(w196) -> ("Bubbler (main).Prep"=w195:bool, "Bubbler (main).Run"=w194:bool, "Bubbler (main).Flow"=w193:dbl, "Dilution"=w192:bool, "Calculated"=w191:u16, "MFC1 flow"=w190:dbl, "MFC2 flow"=w189:dbl, "MFC3 flow"=w188:dbl)
                        n192 = property on="Zn Prep" class="Bool (strict)"("Value"=w195) -> ()  [unwired: 2 in, 2 out]
                        n193 = property on="Zn Run" class="Bool (strict)"("Value"=w194) -> ()  [unwired: 2 in, 2 out]
                        n194 = property on="Zn Flow" class="DigNum (strict)"("Value"=w193) -> ()  [unwired: 2 in, 2 out]
                        n195 = property on="Zn  Dilution" class="Bool (strict)"("Value"=w192) -> ()  [unwired: 2 in, 2 out]
                        n196 = property on="Zn Calculated" class="Ring (strict)"("Value"=w191) -> ()  [unwired: 2 in, 2 out]
                        n197 = property on="Zn MFC1 flow" class="DigNum (strict)"("Value"=w190) -> ()  [unwired: 2 in, 2 out]
                        n198 = property on="Zn MFC2 flow" class="DigNum (strict)"("Value"=w189) -> ()  [unwired: 2 in, 2 out]
                        n199 = property on="Zn MFC3 flow" class="DigNum (strict)"("Value"=w188) -> ()  [unwired: 2 in, 2 out]
                      }
                      frame #7 {
                        n200 = property on="Se bubbler" class="Clust (strict)"() -> ("Value"=w205:T1)  [unwired: 2 in, 2 out]
                        n201 = Unbundle By Name(w205) -> ("Bubbler (main).Prep"=w204:bool, "Bubbler (main).Run"=w203:bool, "Bubbler (main).Flow"=w202:dbl, "Dilution"=w201:bool, "Calculated"=w200:u16, "MFC1 flow"=w199:dbl, "MFC2 flow"=w198:dbl, "MFC3 flow"=w197:dbl)
                        n202 = property on="Se Prep" class="Bool (strict)"("Value"=w204) -> ()  [unwired: 2 in, 2 out]
                        n203 = property on="Se Run" class="Bool (strict)"("Value"=w203) -> ()  [unwired: 2 in, 2 out]
                        n204 = property on="Se Flow" class="DigNum (strict)"("Value"=w202) -> ()  [unwired: 2 in, 2 out]
                        n205 = property on="Se Dilution" class="Bool (strict)"("Value"=w201) -> ()  [unwired: 2 in, 2 out]
                        n206 = property on="Se Calculated" class="Ring (strict)"("Value"=w200) -> ()  [unwired: 2 in, 2 out]
                        n207 = property on="Se MFC1 flow" class="DigNum (strict)"("Value"=w199) -> ()  [unwired: 2 in, 2 out]
                        n208 = property on="Se MFC2 flow" class="DigNum (strict)"("Value"=w198) -> ()  [unwired: 2 in, 2 out]
                        n209 = property on="Se MFC3 flow" class="DigNum (strict)"("Value"=w197) -> ()  [unwired: 2 in, 2 out]
                      }
                    }
                    n210 = property on="is OK?" class="Bool (strict)"("Value"=TRUE ("is OK?")) -> ()  [unwired: 2 in, 2 out]
                  }
                  event Value Change {
                    n211 = event-data() -> ()  [unwired: 1 in, 5 out]
                    n212 = property on="Array" class="Arr (strict)"() -> ("Value"=w206:refnum<vi>[])  [unwired: 2 in, 2 out]
                    n213 = for {
                      tunnel: w206 -> [w208] mode=indexing
                      n214 = control-ref of="Al bubbler"() -> (w207:refnum<vi>)
                      n215 = To More Specific Class(target class=w207, reference=w208) -> (specific class reference=w216:refnum<vi>)  [unwired: 1 in, 1 out]
                      n216 = property class="Clust (strict)"(reference=w216) -> ("Controls[]"=w215:refnum<vi>[])  [unwired: 1 in, 2 out]
                      n217 = control-ref of="Al Run"() -> (w209:refnum<vi>)
                      n218 = Index Array(array=w215, index=1) -> (element=w217:refnum<vi>)
                      n219 = Index Array(array=w215, index=2) -> (element=w213:refnum<vi>)
                      n220 = To More Specific Class(target class=w209, reference=w213) -> (specific class reference=w212:refnum<vi>, error out=w211:errorcluster)  [unwired: 1 in]
                      n221 = property class="Bool (strict)"(reference=w212, error in=w211) -> ("Value"=w210:bool)  [unwired: 2 out]
                      n222 = property class="Ctl"(reference=w217, "Visible"=w210) -> ()  [unwired: 1 in, 2 out]
                    }
                  }
                  event "Cancel": Value Change {
                    n223 = event-data() -> ()  [unwired: 1 in, 5 out]
                  }
                  event Value Change {
                    n224 = event-data() -> ()  [unwired: 1 in, 5 out]
                    n225 = control-ref of="Ga bubbler"() -> (w220:refnum<vi>)
                    n226 = call "dilutionCalcR2.vi"("Clust Refnum"=w220) -> ()
                  }
                  event Value Change {
                    n227 = event-data() -> ()  [unwired: 1 in, 5 out]
                    n228 = control-ref of="Se bubbler"() -> (w221:refnum<vi>)
                    n229 = call "dilutionCalcR2.vi"("Clust Refnum"=w221) -> ()
                  }
                  event Value Change {
                    n230 = event-data() -> ()  [unwired: 1 in, 5 out]
                    n231 = control-ref of="Zn bubbler"() -> (w222:refnum<vi>)
                    n232 = call "dilutionCalcR2.vi"("Clust Refnum"=w222) -> ()
                  }
                }
              }
            }
            frame #2 {
              n233 = property on="is OK?" class="Bool (strict)"() -> ("Value"=w223:bool)  [unwired: 2 in, 2 out]
              n234 = Not(x=w223) -> (.not. x?=w227:bool)
              n235 = Current VI's Path() -> (path=w226:path)
              n236 = call "API_Edit.vi"("Cancel"=w227, "OK"=w223, "VI Path"=w226, "Argument List In"=w224) -> ("Argument List Out"=w225:string[])
            }
          }
          n237 = property class="VI"(reference=w124, "Front Panel.Open"=FALSE ("Front Panel Window:Open"), "FP.Behavior"=T5."Default" ("Front Panel Window:Behavior")) -> (reference out=w125:refnum<vi>)  [unwired: 1 in, 1 out]
          n238 = Close Reference(reference=w125) -> ()  [unwired: 1 in, 1 out]
        }
        frame "Start" {
          n239 = property on="prep_time" class="DigNum (strict)"() -> ("Value"=w232:dbl)  [unwired: 2 in, 2 out]
          n240 = Greater Than 0?(x=w232) -> (x > 0?=w231:bool)
          n241 = Not(x=w229) -> (.not. x?=w228:bool)
          n242 = And(x=w228, y=w231) -> (x .and. y?=w230:bool)
          n243 = case shown="True" w230 {
            frame False {
            }
            frame True {
              n244 = property on="Ga bubbler" class="Clust (strict)"() -> ("Value"=w243:T1)  [unwired: 2 in, 2 out]
              n245 = property on="Zn bubbler" class="Clust (strict)"() -> ("Value"=w237:T1)  [unwired: 2 in, 2 out]
              n246 = property on="Al bubbler" class="Clust (strict)"() -> ("Value"=w244:T2)  [unwired: 2 in, 2 out]
              n247 = property on="In bubbler" class="Clust (strict)"() -> ("Value"=w242:T2)  [unwired: 2 in, 2 out]
              n248 = property on="P gas" class="Clust (strict)"() -> ("Value"=w241:T2)  [unwired: 2 in, 2 out]
              n249 = property on="Se bubbler" class="Clust (strict)"() -> ("Value"=w238:T1)  [unwired: 2 in, 2 out]
              n250 = property on="As gas" class="Clust (strict)"() -> ("Value"=w240:T2)  [unwired: 2 in, 2 out]
              n251 = property on="P bubbler" class="Clust (strict)"() -> ("Value"=w239:T2)  [unwired: 2 in, 2 out]
              n252 = call "Set_V_III.vi"("Se bubbler"=w238, "P bubbler"=w239, "As gas"=w240, "P gas"=w241, "Run Started"=FALSE, "Zn bubbler"=w237, "In bubbler"=w242, "Ga bubbler"=w243, "Al bubbler"=w244) -> ()  [unwired: 3 in]
            }
          }
          n253 = call "Set_Argument.vi"("Enable"=FALSE, "Argument"="run_started", "Argument List In"=w234) -> ("Argument List Out"=w233:string[])
        }
        frame "Run" {
          n254 = stacked-sequence {
            tunnel: w249 -> [_ w254 _ _]
            tunnel: w247 -> [w251 _ _ w276]
            tunnel: w248 -> [_ _ _ w274]
            tunnel: [_ _ _ w275] -> w246
            frame #0 {
              n255 = call "Get_Argument.vi"("Argument"="run_started", "Argument List"=w251) -> ("Enabled"=w250:bool)
              n256 = local write "run started"(w250) -> ()
            }
            frame #1 {
              n257 = property on="prep_time" class="DigNum (strict)"() -> ("Value"=w255:dbl)  [unwired: 2 in, 2 out]
              n258 = Greater Or Equal?(x=w254, y=w255) -> (x >= y?=w253:bool)
              n259 = local write "prep_done"(w253) -> ()
            }
            frame #2 {
              n260 = local read "run started"() -> (w259:bool)
              n261 = property on="Array" class="Arr (strict)"() -> ("Value"=w258:refnum<vi>[])  [unwired: 2 in, 2 out]
              n262 = Not(x=w259) -> (.not. x?=w257:bool)
              n263 = for {
                tunnel: w258 -> [w272] mode=indexing
                tunnel: [w261] -> _ mode=indexing
                shift-right: [w263] -> _
                shift-left: TRUE ("first") -> [w260]
                tunnel: w257 -> [w261]
                n264 = control-ref of="Al bubbler"() -> (w270:refnum<vi>)
                n265 = To More Specific Class(target class=w270, reference=w272) -> (specific class reference=w271:refnum<vi>)  [unwired: 1 in, 1 out]
                n266 = property class="Clust (strict)"(reference=w271) -> ("Value"=w269:T2)  [unwired: 1 in, 2 out]
                n267 = property on="Status Out" class="Str"() -> ("Value"=w265:string)  [unwired: 2 in, 2 out]
                n268 = Unbundle By Name(w269) -> ("Prep"=w268:bool, "Run"=w267:bool, "Active"=w266:bool, "Name"=w262:string)
                n269 = call "flow_strings.vi"("string in"=w265, "is first in?"=w260, "use source?"=w266, "name"=w262, "run source?"=w267, "prep source?"=w268, "is prep?"=w261) -> ("string out"=w264:string, "is first out?"=w263:bool)
                n270 = property on="Status Out" class="Str"("Value"=w264) -> ()  [unwired: 2 in, 2 out]
              }
            }
            frame #3 {
              n271 = property on="run started" class="Bool (strict)"() -> ("Value"=w278:bool)  [unwired: 2 in, 2 out]
              n272 = Not(x=w278) -> (.not. x?=w277:bool)
              n273 = property on="prep_done" class="Bool (strict)"() -> ("Value"=w279:bool)  [unwired: 2 in, 2 out]
              n274 = And(x=w279, y=w277) -> (x .and. y?=w273:bool)
              n275 = case shown="False" w273 {
                selector: w273 -> [_ w281]
                tunnel: w276 -> [w280 w284]
                tunnel: [w280 w283] -> w275
                tunnel: w274 -> [_ w282]
                frame False {
                }
                frame True {
                  n276 = stacked-sequence {
                    tunnel: w282 -> [w286 _]
                    tunnel: w284 -> [_ w297]
                    tunnel: [_ w296] -> w283
                    tunnel: w281 -> [w285 _]
                    frame #0 {
                      n277 = case shown="True" w286 {
                        tunnel: w285 -> [w295 _]
                        frame False {
                          n278 = property on="Ga bubbler" class="Clust (strict)"() -> ("Value"=w293:T1)  [unwired: 2 in, 2 out]
                          n279 = property on="In bubbler" class="Clust (strict)"() -> ("Value"=w292:T2)  [unwired: 2 in, 2 out]
                          n280 = property on="P gas" class="Clust (strict)"() -> ("Value"=w291:T2)  [unwired: 2 in, 2 out]
                          n281 = property on="Al bubbler" class="Clust (strict)"() -> ("Value"=w294:T2)  [unwired: 2 in, 2 out]
                          n282 = property on="Zn bubbler" class="Clust (strict)"() -> ("Value"=w287:T1)  [unwired: 2 in, 2 out]
                          n283 = property on="Se bubbler" class="Clust (strict)"() -> ("Value"=w288:T1)  [unwired: 2 in, 2 out]
                          n284 = property on="As gas" class="Clust (strict)"() -> ("Value"=w290:T2)  [unwired: 2 in, 2 out]
                          n285 = property on="P bubbler" class="Clust (strict)"() -> ("Value"=w289:T2)  [unwired: 2 in, 2 out]
                          n286 = call "Set_V_III.vi"("Se bubbler"=w288, "P bubbler"=w289, "As gas"=w290, "P gas"=w291, "Run Started"=w295, "Zn bubbler"=w287, "In bubbler"=w292, "Ga bubbler"=w293, "Al bubbler"=w294) -> ()  [unwired: 3 in]
                        }
                        frame True {
                        }
                      }
                    }
                    frame #1 {
                      n287 = call "Set_Argument.vi"("Enable"=TRUE, "Argument"="run_started", "Argument List In"=w297) -> ("Argument List Out"=w296:string[])
                    }
                  }
                }
              }
            }
          }
        }
        frame "End" {
        }
        frame "Idle" {
        }
      }
    }
  }
  "Argument List Out" <- w10
  n288 = control-ref of="Ga bubbler"() -> ()  [unwired: 1 out]
  n289 = control-ref of="Al bubbler"() -> ()  [unwired: 1 out]
